vi "make_trans_mat.vi"(3 "Rotation":T1=[[1.0, 0.0, 0.0], [0.0, 1.0, 0.0], [0.0, 0.0, 1.0]], 5 "Translation":T1=[[0.0], [0.0], [0.0]]) -> (1 "Transform":T1)   [LabVIEW 2013]
uses:
  <vilib>/Analysis/Matrix/Datatypes/RealMatrix.ctl
  <vilib>/Analysis/Matrix/Numeric/Conversions/Array To Matrix - RA.vi
  <vilib>/Analysis/Matrix/NI_Matrix.lvlib
panel:
  # "Create 4x4 linear homogenous transform from rotation and translation parts."
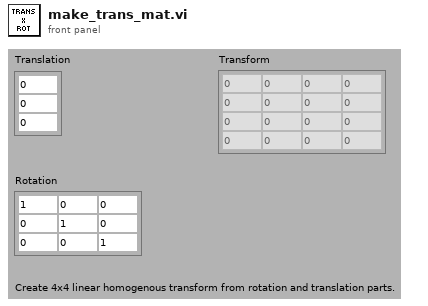
[diagram p1: front panel]
types:
  T1 = typedef "NI_Matrix.lvlib/RealMatrix.ctl" = dbl[][]
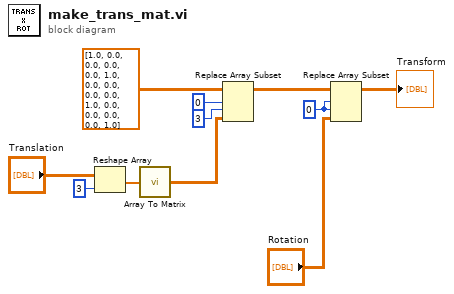
[diagram p0: block diagram]
diagram:
  w11 = 0 ("disabled index (row)")
  n1 = Reshape Array("Translation", 3 ("dimension size")) -> (w2:dbl[])
  n2 = call-poly <vilib>:"Array To Matrix.vi"("Real 1D Array"=w2) -> ("Real Matrix (Column Vector)"=w1:T1)
  n3 = Replace Array Subset(array=T1 [[1.0, 0.0, 0.0, 0.0], [0.0, 1.0, 0.0, 0.0], [0.0, 0.0, 1.0, 0.0], [0.0, 0.0, 0.0, 1.0]] ("Translation"), new element=w1, index (row)=0 ("disabled index (row)"), index (col)=3 ("disabled index (col)")) -> (w8:T1)
  n4 = Replace Array Subset(array=w8, new element="Rotation", index (row)=w11, index (col)=w11) -> (→"Transform":T1)
